vi "SPD.KC705 Test.vi"(8 "Error In":errorcluster, 11 "SPD.Stand Ctrl in":T1) -> (0 "Error Out":errorcluster, 1 "ok":bool, 2 "report":string, 3 "SPD.Stand Ctrl out":T1)   [LabVIEW 2018]
uses:
  typedefs/SPD.Stand Ctrl.ctl
  Instruments/SPD HID Interface/hidSPDLibForLabView/LibVIs/hidSPD Controls/hidSPD Device Session.ctl
  Instruments/KC705 DevBoard/typedefs/DevB.Session.ctl
  Instruments/KeySight 53230A/typedefs/FreqC.Session.ctl
  Instruments/KeySight 8164B/KeySight 8164B LAN InstrLib/typedefs/KeySight 8164B control.ctl
  Instruments/LeCroy SDA830/typedefs/LeCroy.Session.ctl
  <vilib>/measure/mamon.llb/Trigger Detection for 1 Channel.vi
  Instruments/LeCroy SDA830/LeCroy SDA830 API/Read/LeCroy.Read Single Waveform.vi
  <vilib>/measure/NI_MAPro.lvlib
  Instruments/SPD HID Interface/hidSPDLibForLabView/hidSPDLibForLabView.lvlib
  Instruments/KeySight 8164B/KeySight 8164B LAN InstrLib.lvlib
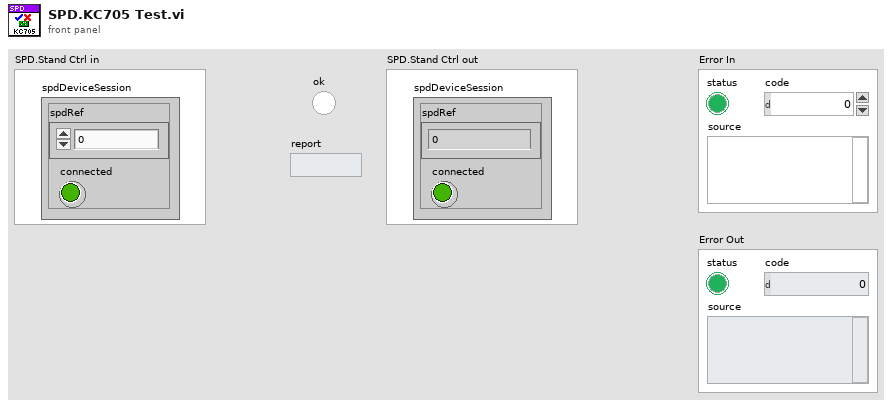
[diagram p1: front panel]
types:
  T1 = typedef "SPD.Stand Ctrl.ctl" = cluster{"spdDeviceSession":T2, "DevBSession":T3, "FreqCSession":T4, "8164BSession":T5, "LeCroySession":T6}
  T2 = typedef "hidSPDLibForLabView.lvlib/hidSPD Device Session.ctl" = cluster{"spdRef":u64, "connected":bool}
  T3 = typedef "DevB.Session.ctl" = cluster{"DevBRef":refnum<visa-resource-name>, "connected":bool}
  T4 = typedef "FreqC.Session.ctl" = cluster{"FreqCRef":refnum<visa-resource-name>, "timeout":dbl, "connected":bool}
  T5 = typedef "KeySight 8164B LAN InstrLib.lvlib/KeySight 8164B control.ctl" = cluster{"Connection ID":refnum<k5>, "Connected":bool, "Info":string, "Slots Info":string[]}
  T6 = typedef "LeCroy.Session.ctl" = cluster{"LeCroySession":refnum<visa-resource-name>, "connected":bool}
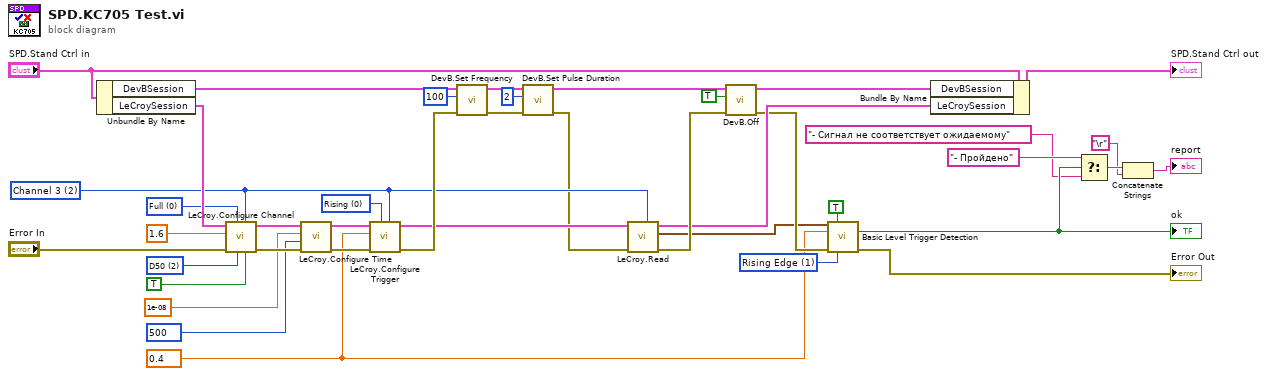
[diagram p0: block diagram]
diagram:
  w4 = u16 1 items=["Falling Edge", "Rising Edge"] ("trigger slope")
  w21 = u16 0 items=["Rising", "Falling"] ("Trigger Slope")
  w5 = 0.4 ("Trigger Level")
  w23 = 500 items=["50"=50, "100"=100, "250"=250, "500"=500, "1000"=1000, "2500"=2500, "5K"=5000, "10K"=10000, "25K"=25000, "50K"=50000, "100K"=100000, "250K"=250000, "500K"=500000, "1M"=1000000, "2M"=2000000, "2.5M"=2500000, "5M"=5000000, "10M"=10000000, "25M"=25000000, "50M"=50000000, "100M"=100000000] ("Sample Points")
  w28 = u16 2 items=["A1M", "D1M", "D50", "Ground", "DC", "AC"] ("Coupling")
  w30 = u16 0 items=["Full", "20MHZ", "25MHZ", "200MHZ", "250MHZ", "1GHZ", "3GHZ", "4GHZ"] ("Bandwidth")
  w15 = u16 2 items=["Channel 1", "Channel 2", "Channel 3", "Channel 4"] ("Channel")
  n1 = Unbundle By Name("SPD.Stand Ctrl in") -> ("DevBSession"=w18:T3, "LeCroySession"=w32:T6)
  n2 = call "LeCroy.Configure Channel.vi"("Enable"=TRUE, "Channel"=w15, "Coupling"=w28, "Bandwidth"=w30, "Error In"="Error In", "Vertical Range"=1.6, "LeCroy.Session in"=w32) -> ("Error Out"=w25:errorcluster, "LeCroy.Session out"=w26:T6)  [unwired: 3 in]
  n3 = call "LeCroy.Configure Time.vi"("Error In"=w25, "Sample Points"=w23, "Timebase"=1e-08, "LeCroy.Session in"=w26) -> ("Error Out"=w20:errorcluster, "LeCroy.Session out"=w22:T6)  [unwired: 6 in]
  n4 = call "LeCroy.Configure Trigger.vi"("Trigger Source"=w15, "Trigger Slope"=w21, "Error In"=w20, "Trigger Level"=w5, "LeCroy.Session in"=w22) -> ("Error Out"=w19:errorcluster, "LeCroy.Session out"=w16:T6)  [unwired: 5 in]
  n5 = call "DevB.Set Frequency.vi"("error in (no error)"=w19, "Frequency"=100, "DevB Session in"=w18) -> ("error out"=w17:errorcluster, "DevB Session out"=w34:T3)  [unwired: 7 in]
  n6 = call "DevB.Set Pulse Duration.vi"("error in (no error)"=w17, "Pulse Duration"=2, "DevB Session in"=w34) -> ("error out"=w14:errorcluster, "DevB Session out"=w13:T3)  [unwired: 7 in]
  n7 = call-poly "LeCroy.Read.vi"("Source"=w15, "Error In"=w14, "LeCroy.Session in"=w16) -> ("Error Out"=w11:errorcluster, "Waveform Data"=w7:waveform(dbl), "LeCroy.Session out"=w9:T6)  [unwired: 6 in]
  n8 = call "DevB.Off.vi"("error in (no error)"=w11, "off"=TRUE, "DevB Session in"=w13) -> ("error out"=w8:errorcluster, "DevB Session out"=w10:T3)  [unwired: 7 in]
  n9 = call-poly <vilib>:"Basic Level Trigger Detection.vi"("signal in"=w7, "reset"=TRUE, "level"=w5, "error in (no error)"=w8, "trigger slope"=w4) -> ("trigger detected?"=w3:bool, "error out"=→"Error Out":errorcluster)  [unwired: 8 in, 1 out]
  "ok" <- w3
  n10 = Bundle By Name(cluster="SPD.Stand Ctrl in", "DevBSession"=w10, "LeCroySession"=w9) -> (→"SPD.Stand Ctrl out":T1)
  n11 = Select(t="- Пройдено" ("report"), s=w3, f="- Сигнал не соответствует ожидаемому") -> (s? t:f=w38:string)
  n12 = Concatenate Strings(w38, "\r") -> (→"report":string)
